vi "GratingSelect.vi"(8 "error in (no error)":errorcluster, 10 "Current Grating":u8=1, 11 "VISA resource name":refnum<visa-resource-name>) -> (0 "error out":errorcluster, 2 "Command not accepted":bool, 3 "VISA resource name out":refnum<visa-resource-name>)   [LabVIEW 2017, in "Spectral Products CM110.lvlib"]
uses:
  Spectral Products CM110.lvlib
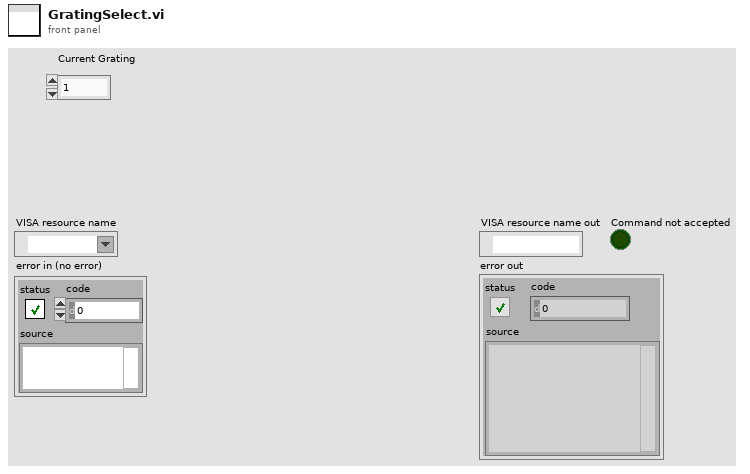
[diagram p1: front panel]
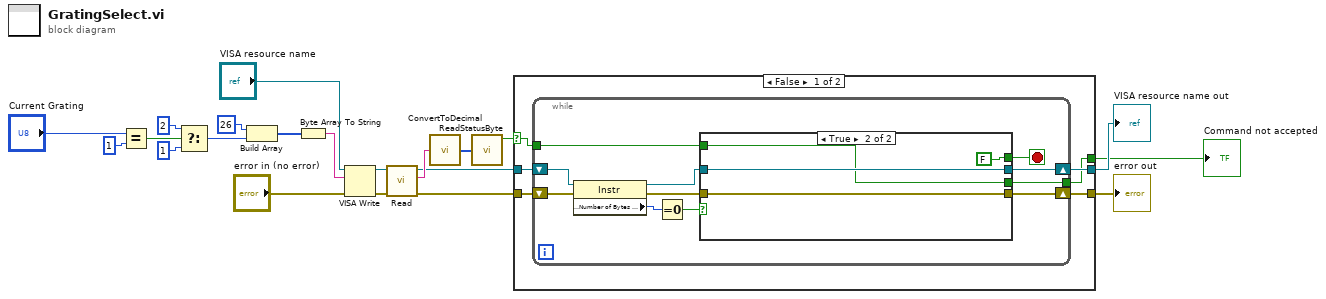
[diagram p0: block diagram]
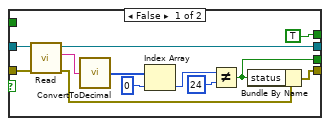
[diagram p2: hidden frame]
diagram:
  n1 = Equal?(x="Current Grating", y=u8 1) -> (x = y?=w10:bool)
  n2 = Select(t=u8 2, s=w10, f=u8 1) -> (s? t:f=w7:u8)
  n3 = Build Array(u8 26, w7) -> (w17:u8[])
  n4 = Byte Array To String(unsigned byte array=w17) -> (string=w16:string)
  n5 = VISA Write(VISA resource name="VISA resource name", write buffer=w16, error in (no error)="error in (no error)") -> (VISA resource name out=w14:refnum<visa-resource-name>, error out=w13:errorcluster)  [unwired: 1 out]
  n6 = call "Read.vi"("error in (no error)"=w13, "VISA Refnum in"=w14) -> ("error out"=w4:errorcluster, "read buffer"=w19:string, "VISA Refnum out"=w5:refnum<visa-resource-name>)  [unwired: 6 in, 1 out]
  n7 = call "ConvertToDecimal.vi"("read buffer"=w19) -> ("unsigned byte array"=w15:u8[])
  n8 = call "ReadStatusByte.vi"("unsigned byte array"=w15) -> ("Command not accepted"=w6:bool)  [unwired: 4 in, 5 out]
  n9 = case shown="False" w6 {
    selector: w6 -> [w22 w55]
    tunnel: w5 -> [w27 w57]
    tunnel: w4 -> [w26 w56]
    tunnel: [w25 w57] -> w3
    tunnel: [w24 w56] -> w2
    tunnel: [w23 w55] -> w1
    frame False {
      n10 = while {
        shift-right: [w31] -> w25
        shift-left: w27 -> [w38]
        shift-right: [w30] -> w24
        shift-left: w26 -> [w37]
        tunnel: [w29] -> w23
        tunnel: w22 -> [w28]
        stop <- w36 stop-if-true
        n11 = property class="Instr"(reference=w38, error in=w37) -> (reference out=w35:refnum<visa-resource-name>, error out=w34:errorcluster, "Serial Settings:Number of Bytes at Serial Port"=w33:u32)
        n12 = Equal To 0?(x=w33) -> (x = 0?=w32:bool)
        n13 = case shown="True" w32 {
          tunnel: [TRUE FALSE] -> w36
          tunnel: w35 -> [w50 w53]
          tunnel: w34 -> [w49 w52]
          tunnel: [w42 w53] -> w31
          tunnel: [w40 w52] -> w30
          tunnel: [w39 w51] -> w29
          tunnel: w28 -> [_ w51]
          frame False {
            n14 = call "Read.vi"("error in (no error)"=w49, "VISA Refnum in"=w50) -> ("error out"=w41:errorcluster, "read buffer"=w48:string, "VISA Refnum out"=w42:refnum<visa-resource-name>)  [unwired: 6 in, 1 out]
            n15 = call "ConvertToDecimal.vi"("read buffer"=w48) -> ("unsigned byte array"=w47:u8[])
            n16 = Index Array(array=w47, index=0) -> (element=w45:u8)
            n17 = Not Equal?(x=w45, y=u8 24) -> (x != y?=w39:bool)
            n18 = Bundle By Name(cluster=w41, "status"=w39) -> (w40:errorcluster)
          }
          frame True {
          }
        }
      }
    }
    frame True {
    }
  }
  "VISA resource name out" <- w3
  "error out" <- w2
  "Command not accepted" <- w1
